vi "Tree Edit.vi"(8 "error in (no error)":errorcluster, 11 "Tree DVR in":refnum<data-value>) -> (0 "error out":errorcluster, 3 "Tree DVR out":refnum<data-value>)   [LabVIEW 2012, in "MDSplus.lvlib"]
doc: "Open the tree for editing."
uses:
  <vilib>/MDSplus/Library/MDSplus.lvlib
  <vilib>/MDSplus/Classes/Tree_Class/Tree.lvclass
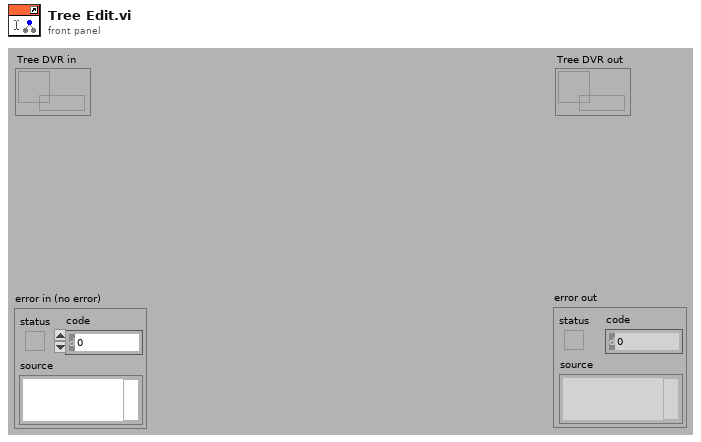
[diagram p1: front panel]
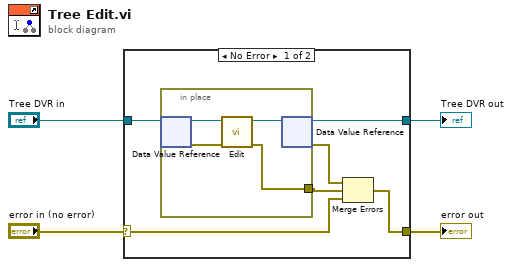
[diagram p0: block diagram]
diagram:
  n1 = case shown="No Error" "error in (no error)" {
    selector: "error in (no error)" -> [w9 w16]
    tunnel: "Tree DVR in" -> [w10 w15]
    tunnel: [w7 w16] -> w4
    tunnel: [w6 w15] -> w1
    frame No Error {
      n2 = in-place {
        in-place-border: [w12] -> w5
        n3 = in-place-dvr #1(w10) -> (w14:refnum<class "Tree.lvclass">, w11:errorcluster)
        n4 = call-dynamic "Edit.vi"("error in (no error)"=w11, "Tree in"=w14) -> ("error out"=w12:errorcluster, "Tree out"=w13:refnum<class "Tree.lvclass">)  [unwired: 8 in]
        n5 = in-place-dvr #1(w13) -> (w6:refnum<data-value>, w8:errorcluster)
      }
      n6 = Merge Errors(w8, w5, w9) -> (w7:errorcluster)
    }
    frame Error {
    }
  }
  "error out" <- w4
  "Tree DVR out" <- w1
